vi "Latch onto Controller.vi"(8 "error in":errorcluster) -> ()   [LabVIEW 2017]
doc: "This VI executes continuously carrying out the current operation and responding to updates or new operations. It will often contain the timing or control code that is difficult to place directly in TeleOp. This VI generally opens all sensors and motors and isolates the rest of the robot code from knowing how the operations are carried out."
uses:
  <vilib>/Rock Robotics/WPI/Framework/Completion Status.ctl
  Latch onto Setpoints.ctl
  Latch onto Operations.ctl
  <vilib>/Rock Robotics/SystemInterfaces/DIO/FPGA_DIOPWMChannel.ctl
  <vilib>/Rock Robotics/WPI/MotorControl/WPI_MotorControlOpen SPARK.vi
  <vilib>/Rock Robotics/Network Tables/NT Write Number.vi
panel:
  in  "Interactive Values":T1
  out "Current\nCmd":string
  in  "Buttons":cluster{"Execute Cmd":bool, "Abort Cmd":bool}
  out "Command Timing":cluster{"Start Time (ms)":u32, "Iterations":i32}
  out "Status":T3
  # "Tip: It may be helpful to observe inputs and sensor values.\nYou may also want to display tuning or debugging controls."
  # "Interactive Command: You may fill in the settings for a command\nand schedule it with the Execute button. You can observe and abort\nany command while fine tuning the code for the controller."
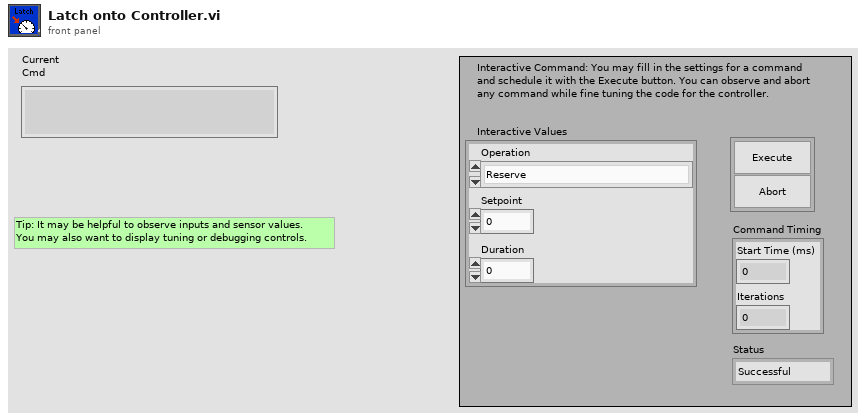
[diagram p1: front panel]
types:
  T1 = typedef "Latch onto Setpoints.ctl" = cluster{"Operation":T2, "Setpoint":dbl, "Duration":dbl}
  T2 = typedef "Latch onto Operations.ctl" = enum16{"Reserve", "Read Current", "Immediate", "Latch"}
  T3 = typedef "Completion Status.ctl" = enum16{"Successful", "Aborted", "Incomplete"}
  T4 = typedef "FPGA_DIOPWMChannel.ctl" = enum8{"PWM 0", "PWM 1", "PWM 2", "PWM 3", "PWM 4", "PWM 5", "PWM 6", "PWM 7", "PWM 8", "PWM 9", "PWM MXP 0", "PWM MXP 1", "PWM MXP 2", "PWM MXP 3", "PWM MXP 4", "PWM MXP 5", "PWM MXP 6", "PWM MXP 7", "PWM MXP 8", "PWM MXP 9", "Invalid"}
  T5 = typedef "WPI_MotorControlDeviceRef.ctl" = cluster{"DeviceStatus":errorcluster, "Type":T6, "PWM":cluster{"PWM Channel":T4, "DeadBand":T7}, "CAN":cluster{"Device Number":u8, "SetOutput VI Ref":variant, "GetOutput VI Ref":variant, "Enable VI Ref":variant, "Disable VI Ref":variant, "Data":variant}, "Invert":bool, "DIO PWM":cluster{"PWM \"Enable\" Channel":T4, "DIOChannel":T8, "PWM Rate":dbl}}
  T6 = typedef "WPI_MotorControlType.ctl" = enum16{"PWM", "CAN", "DIO PWM"}
  T7 = typedef "WPI_PWMDeadband.ctl" = cluster{"Name":string, "maxPositivePwm":i32, "minPositivePwm":i32, "centerPwm":i32, "maxNegativePwm":i32, "minNegativePwm":i32, "angularRange":u16}
  T8 = typedef "FPGA_DIOChannel.ctl" = enum8{"DIO 0", "DIO 1", "DIO 2", "DIO 3", "DIO 4", "DIO 5", "DIO 6", "DIO 7", "DIO 8", "DIO 9", "DIO MXP 0", "DIO MXP 1", "DIO MXP 2", "DIO MXP 3", "DIO MXP 4", "DIO MXP 5", "DIO MXP 6", "DIO MXP 7", "DIO MXP 8", "DIO MXP 9", "DIO MXP 10", "DIO MXP 11", "DIO MXP 12", "DIO MXP 13", "DIO MXP 14", "DIO MXP 15", "SPI Port CS1", "SPI Port CS2", "SPI Port CS3", "SPI Port MISO", "SPI Port MOSI", "Invalid"}
  T9 = typedef "Command Status Info.ctl" = cluster{"Name":string, "Status":T3, "notifier out":T10}
  T10 = typedef "Completion Notifier.ctl" = refnum<notifier>
  T11 = cluster{"Current Command":T1, "Command Timing":cluster{"Start Time (ms)":u32, "Iterations":i32}, "Command Arguments":cluster{"Command Info":T9, "Description":string, "Default Command":T1, "queue out":refnum<queue>, "Subsystem Name":string}}
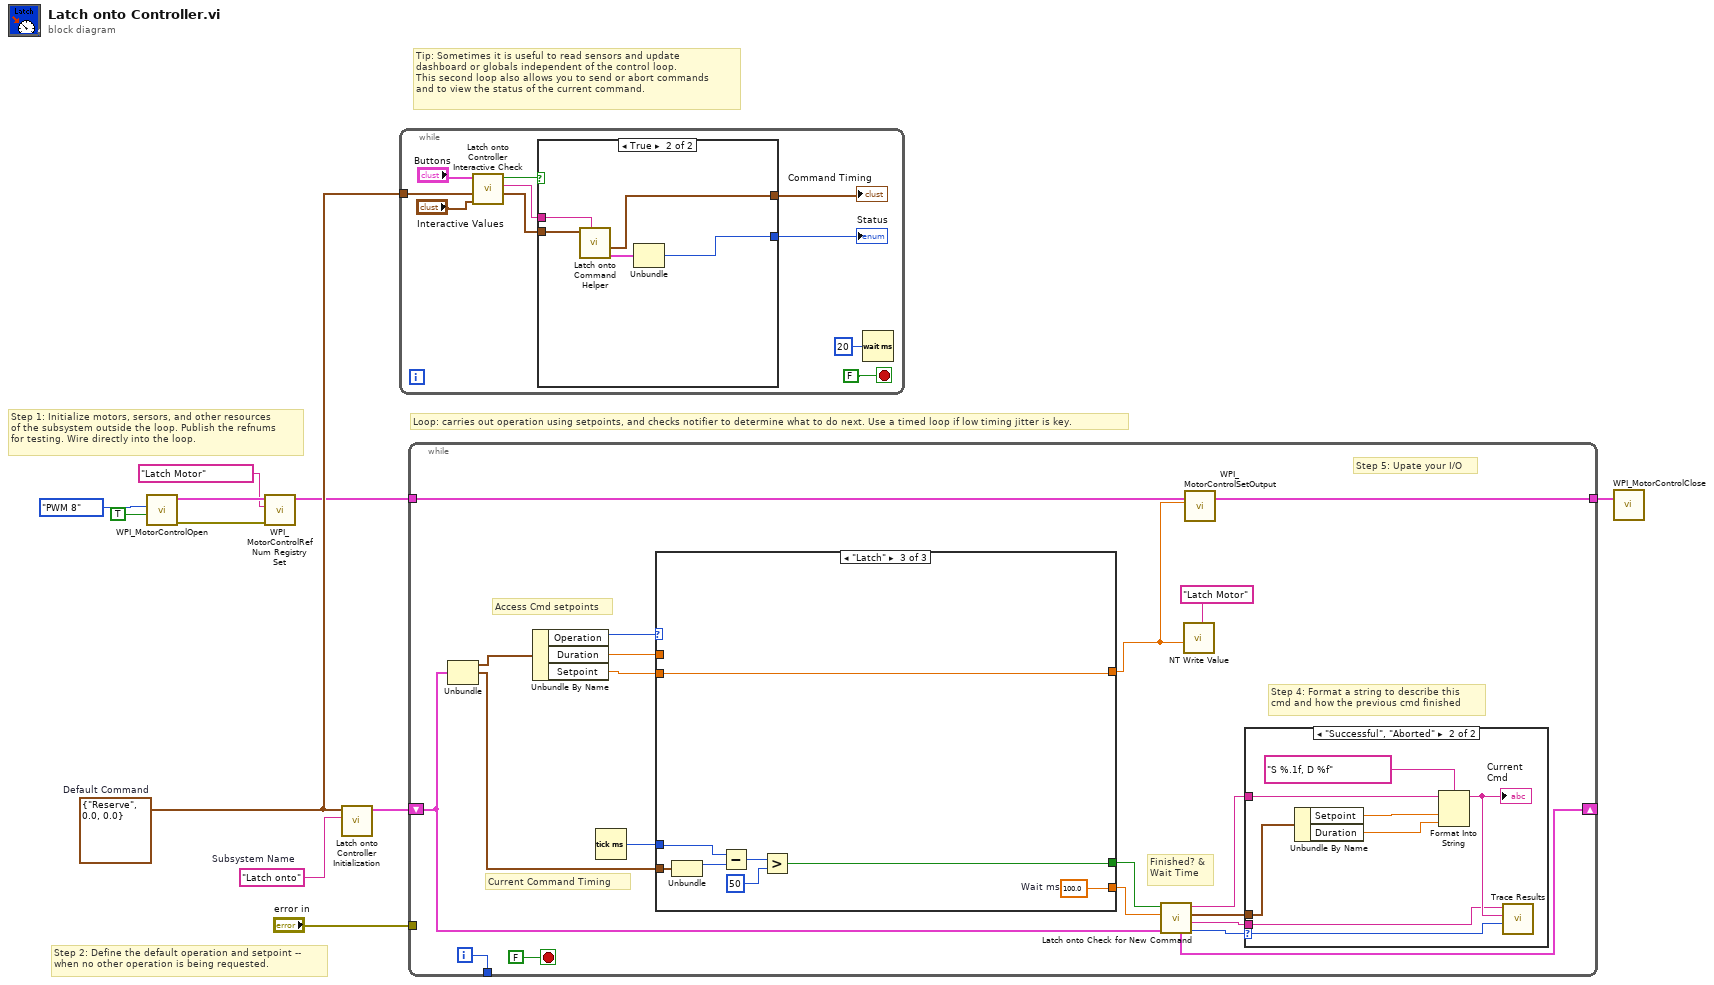
[diagram p0: block diagram]
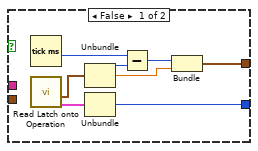
[diagram p2: hidden frame]
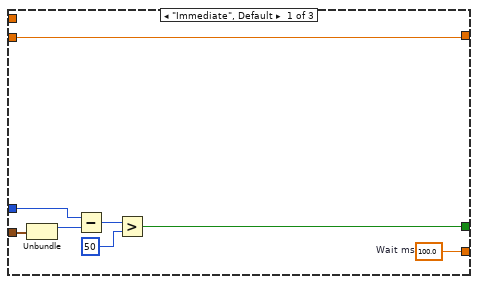
[diagram p4: hidden frame]
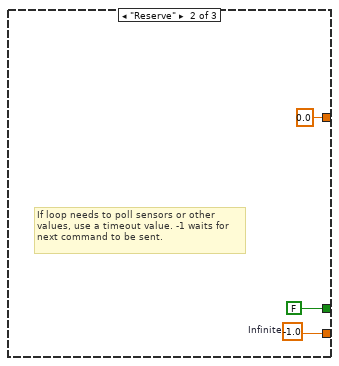
[diagram p5: hidden frame]
diagram:
  w8 = T1 {"Operation"=enum."Reserve", "Setpoint"=0.0, "Duration"=0.0}  # Default Command
  w9 = "Latch onto"  # Subsystem Name
  # "Tip: Sometimes it is useful to read sensors and update\ndashboard or globals independent of the control loop.\nThis second loop also allows you to send or abort commands\nand to view the status of the current command."
  # "Step 2: Define the default operation and setpoint --\nwhen no other operation is being requested."
  # "Step 1: Initialize motors, sersors, and other resources\nof the subsystem outside the loop. Publish the refnums\nfor testing. Wire directly into the loop."
  # "Loop: carries out operation using setpoints, and checks notifier to determine what to do next. Use a timed loop if low timing jitter is key."
  n1 = call-poly <vilib>:"WPI_MotorControlOpen.vi"("Eliminate Deadband"=TRUE, "PWM Channel"=FPGA_DIOPWMChannel."PWM 8") -> ("error out"=w5:errorcluster, "MotorControlDeviceRef"=w4:T5)  [unwired: 8 in]
  n2 = call <vilib>:"WPI_MotorControlRefNum Registry Set.vi"("error in (no error)"=w5, "refnum name"="Latch Motor", "MotorControlDevRef"=w4) -> ("MotorControlDevRef"=w1:T5)  [unwired: 7 in, 1 out]
  n3 = call "Latch onto Controller Initialization.vi"("Subsystem Name"=w9, "Default Command"=w8) -> ("Current Command"=w10:T11)  [unwired: 9 in]
  n4 = while {
    tunnel: w8 -> [w18]
    stop <- FALSE stop-if-true
    n5 = call "Latch onto Controller Interactive Check.vi"("Interactive Command in"="Interactive Values", "Default Command"=w18, "Buttons"="Buttons") -> ("Interactive Command out"=w15:T1, "Trace String"=w16:string, "Schedule"=w17:bool)  [unwired: 6 in]
    n6 = case shown="True" w17 {
      tunnel: [w29 w34] -> w14
      tunnel: w15 -> [_ w32]
      tunnel: [w25 w30] -> w13
      tunnel: w16 -> [_ w33]
      frame False {
        n7 = Tick Count (ms)() -> (millisecond timer value=w24:u32)
        n8 = call "Read Latch onto Operation.vi"() -> ("Command Info"=w22:T9, "SubSystem Data"=w23:T1)  [unwired: 9 in, 1 out]
        n9 = Unbundle(w23) -> ("Operation"=w28:T2, "Setpoint"=w26:dbl)  [unwired: 1 out]
        n10 = Unbundle(w22) -> ("Status"=w29:T3)  [unwired: 2 out]
        n11 = Subtract(x=w24, y=w28) -> (x-y=w27:u32)
        n12 = Bundle(w27, "Setpoint"=w26) -> (w25:cluster{u32, "Setpoint":dbl})  [unwired: 1 in]
      }
      frame True {
        n13 = call "Latch onto Command Helper.vi"("Description"=w33, "SubSystem Data"=w32) -> ("Command Info Out"=w31:T9, "Command Timing"=w30:cluster{"Start Time (ms)":u32, "Iterations":i32})  [unwired: 7 in, 1 out]
        n14 = Unbundle(w31) -> ("Status"=w34:T3)  [unwired: 2 out]
      }
    }
    "Status" <- w14
    "Command Timing" <- w13
    n15 = Wait (ms)(milliseconds to wait=u32 20) -> ()  [unwired: 1 out]
  }
  n16 = while {
    shift-right: [w46] -> _
    shift-left: w10 -> [w39]
    tunnel: [w53] -> _
    tunnel: "error in" -> [_]
    tunnel: [w36] -> w2
    tunnel: w1 -> [w37]
    i -> [w53]
    stop <- FALSE stop-if-true
    # "Step 5: Upate your I/O"
    # "Step 4: Format a string to describe this\ncmd and how the previous cmd finished"
    # "Current Command Timing"
    # "Access Cmd setpoints"
    # "Finished? &\nWait Time"
    n17 = Unbundle(w39) -> ("Current Command"=w52:T1, "Command Timing"=w48:cluster{"Start Time (ms)":u32, "Iterations":i32})  [unwired: 1 out]
    n18 = Unbundle By Name(w52) -> ("Operation"=w51:T2, "Duration"=w50:dbl, "Setpoint"=w47:dbl)
    n19 = Tick Count (ms)() -> (millisecond timer value=w49:u32)
    n20 = case shown="\"Latch\"" w51 {
      tunnel: [w70 w73 w74] -> w44
      tunnel: [w64 FALSE ("ignore previous (F)") w75] -> w45
      tunnel: w48 -> [w66 _ w77]
      tunnel: w50 -> [_ _ _]
      tunnel: w49 -> [w65 _ w76]
      tunnel: w47 -> [w63 _ w81]
      tunnel: [w63 0.0 ("Setpoint") w81] -> w38
      frame "Immediate", Default {
        w70 = 100.0  # Wait ms
        n21 = Unbundle(w66) -> ("Start Time (ms)"=w69:u32)  [unwired: 1 out]
        n22 = Subtract(x=w65, y=w69) -> (x-y=w68:u32)
        n23 = Greater?(x=w68, y=u8 50 ("Left Motor")) -> (0:w64:bool)
      }
      frame "Reserve" {
        w73 = -1.0  # Infinite
        # "If loop needs to poll sensors or other\nvalues, use a timeout value. -1 waits for\nnext command to be sent."
      }
      frame "Latch" {
        w74 = 100.0  # Wait ms
        n24 = Unbundle(w77) -> ("Start Time (ms)"=w80:u32)  [unwired: 1 out]
        n25 = Subtract(x=w76, y=w80) -> (x-y=w79:u32)
        n26 = Greater?(x=w79, y=u8 50 ("Left Motor")) -> (0:w75:bool)
      }
    }
    n27 = call "Latch onto Check for New Command.vi"("Current Command"=w39, "Wait time (ms)"=w44, "Finished?"=w45) -> ("Completion"=w40:T3, "Subsystem Name"=w41:string, "Current Command"=w42:T1, "Initial Trace String"=w43:string, "NextCommand"=w46:T11)  [unwired: 4 in]
    n28 = call-poly <vilib>:"NT Write Value.vi"("Numeric"=w38, "Name"="Latch Motor") -> ()  [unwired: 9 in, 1 out]
    n29 = call <vilib>:"WPI_MotorControlSetOutput.vi"("Output"=w38, "MotorControlDevRef"=w37) -> ("MotorControlDevRef"=w36:T5)  [unwired: 7 in, 2 out]
    n30 = case shown="\"Successful\", \"Aborted\"" w40 {
      selector: w40 -> [_ w62]
      tunnel: w43 -> [_ w58]
      tunnel: w42 -> [_ w59]
      tunnel: w41 -> [_ w55]
      frame "Incomplete", Default {
        # "Continuing current command"
      }
      frame "Successful", "Aborted" {
        # "Report and setup for next command"
        n31 = Unbundle By Name(w59) -> ("Setpoint"=w61:dbl, "Duration"=w56:dbl)
        n32 = Format Into String(format string="S %.1f, D %f", initial string=w58, w61, w56) -> (resulting string=w57:string)  [unwired: 1 in, 1 out]
        "Current\nCmd" <- w57
        n33 = call <vilib>:"Trace Results.vi"("Status of previous command"=w62, "Description"=w57, "Subsystem"=w55) -> ()  [unwired: 9 in]
      }
    }
  }
  n34 = call <vilib>:"WPI_MotorControlClose.vi"("MotorControlDevRef"=w2) -> ()  [unwired: 10 in, 1 out]
